vi "Write Reader.vi"(8 "error in (no error)":errorcluster, 10 "Reader":refnum<k24>, 11 "ADOResult in":refnum<class "ADOResult.lvclass">) -> (0 "error out":errorcluster, 3 "ADOResult out":refnum<class "ADOResult.lvclass">)   [LabVIEW 2020, in "ORM_ADONet.lvlib" / "ADOResult.lvclass"]
uses:
  ADOResult.lvclass
  System.Data
  ADOResult.lvclass/ADOResult.ctl
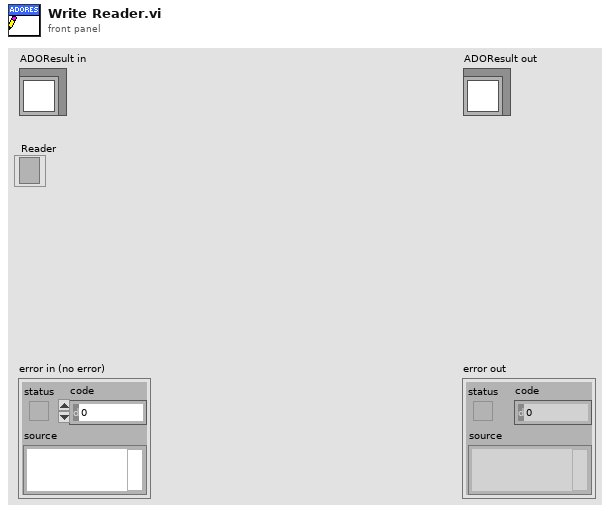
[diagram p1: front panel]
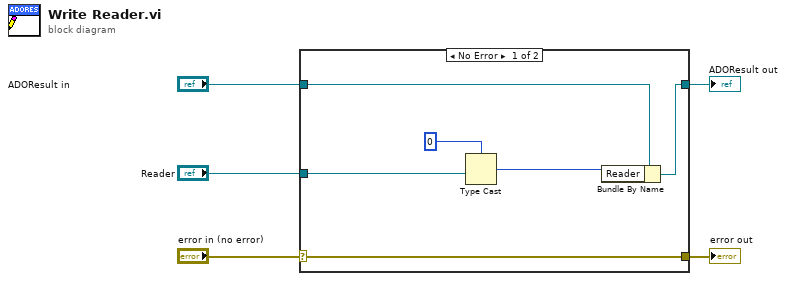
[diagram p0: block diagram]
diagram:
  n1 = case shown="No Error" "error in (no error)" {
    selector: "error in (no error)" -> [w11 w12]
    tunnel: [w11 w12] -> w4
    tunnel: [w9 w13] -> w2
    tunnel: "ADOResult in" -> [w10 w13]
    tunnel: "Reader" -> [w8 _]
    frame No Error {
      n2 = Type Cast(type=u64 0 ("Reader"), x=w8) -> (*(type *) &x=w6:u64)
      n3 = Bundle By Name(cluster=w10, "Reader"=w6) -> (w9:refnum<class "ADOResult.lvclass">)
    }
    frame Error {
    }
  }
  "error out" <- w4
  "ADOResult out" <- w2
